vi "CH_LM Callback USBStreamingData.vi"(4 "User Parameter":variant, 5 "Event Data":T2, 6 "Control Ref":refnum<k7>, 7 "Event Common Data":T3) -> ()   [LabVIEW 2017, in "CH_LM.lvlib"]
doc: "This ActiveX callback VI is executed every time the corresponding ActiveX StreamData event occurs.\n\nThe event name together with the event data is written into a queue which is derived from a FGV (CH_SSIM Global Event Queues.vi). The queue is read from the CH_SSIM Streaming Read Data.vi.\n\n<B>Information:</B> ActiveX events with no corresponding combination of serial number and valid queue reference in the FGV are lost."
uses:
  CH_LM.lvlib
  CH_LM Event Cluster.ctl
  CH_LM Action Enumeration.ctl
  CH_LM_App/CH_LM Globals Debug-Status.vi
  CH_LM App.lvlib
panel:
  in  "CH_LM Event Cluster":T1
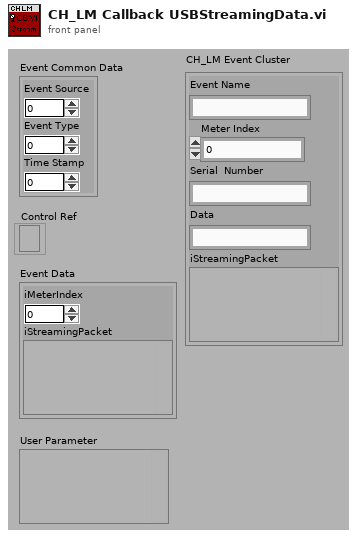
[diagram p1: front panel]
types:
  T1 = typedef "CH_LM.lvlib/CH_LM Event Cluster.ctl" = cluster{"Event Name":string, "Meter Index":i32, "Serial  Number":string, "Data":string, "iStreamingPacket":variant}
  T2 = cluster{"iMeterIndex":i16, "iStreamingPacket":variant}
  T3 = cluster{"Event Source":i32, "Event Type":u32, "Time Stamp":u32}
  T4 = typedef "CH_LM.lvlib/CH_LM Action Enumeration.ctl" = enum16{"add", "read", "read by serial", "set", "remove", "delete", "Clear Shift-Register", ""}
  T5 = typedef "CH_LM.lvlib/CH_LM Meter Info.ctl" = cluster{"Meter Index":i32, "Serial Number":string, "Queue Cluster":T6, "Data Header":bool, "Data Tokens":T7[]}
  T6 = typedef "CH_LM.lvlib/CH_LM Queue Cluster.ctl" = cluster{"Streaming Queue":refnum<queue>, "Asynch Notifier":refnum<notifier>}
  T7 = typedef "CH_LM.lvlib/CH_LM Data Token.ctl" = enum16{"Raw data", "Quad distance", "Formated data", "Unit", "Pulse period", "Flags", "Sequence ID"}
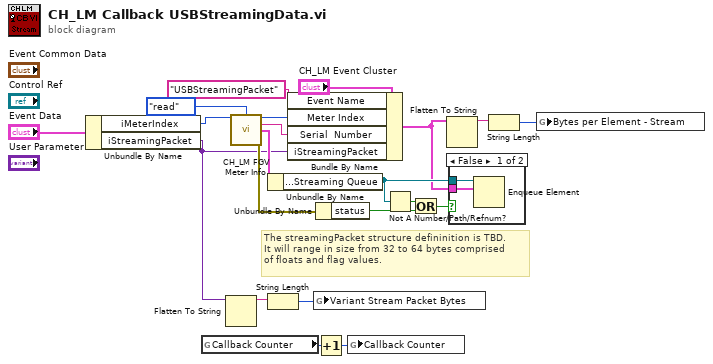
[diagram p0: block diagram]
diagram:
  # "The streamingPacket structure defininition is TBD.\nIt will range in size from 32 to 64 bytes comprised\nof floats and flag values."
  n1 = Unbundle By Name("Event Data") -> ("iMeterIndex"=w9:i16, "iStreamingPacket"=w8:variant)
  n2 = global read "CH_LM Globals Debug-Status.vi" "Callback Counter"() -> (w2:i32)
  n3 = Flatten To String(anything=w8) -> (data string=w7:string)  [unwired: 3 in, 2 out]
  n4 = call "CH_LM FGV Meter Info.vi"("Meter Index"=w9, "Action (read)"=CH_LM_Action_Enumeration."read") -> ("Meter Index out"=w12:i32, "Serial Number out"=w11:string, "Meter Info"=w19:T5, "error out"=w18:errorcluster)  [unwired: 3 in, 7 out]
  n5 = Unbundle By Name(w19) -> ("Queue Cluster.Streaming Queue"=w20:refnum<queue>)
  n6 = String Length(string=w7) -> (length=w6:i32)
  n7 = Bundle By Name(cluster="CH_LM Event Cluster", "Event Name"="USBStreamingPacket", "Meter Index"=w12, "Serial  Number"=w11, "iStreamingPacket"=w8) -> (w3:T1)
  n8 = global write "CH_LM Globals Debug-Status.vi" "Variant Stream Packet Bytes"(w6) -> ()
  n9 = Unbundle By Name(w18) -> ("status"=w14:bool)
  n10 = Increment(x=w2) -> (x+1=w1:i32)
  n11 = global write "CH_LM Globals Debug-Status.vi" "Callback Counter"(w1) -> ()
  n12 = Not A Number/Path/Refnum?(number/path/refnum=w20) -> (NaN/Path/Refnum?=w15:bool)
  n13 = Or(x=w15, y=w14) -> (x .or. y?=w13:bool)
  n14 = Flatten To String(anything=w3) -> (data string=w5:string)  [unwired: 3 in, 2 out]
  n15 = case shown="False" w13 {
    tunnel: w3 -> [w23 _]
    tunnel: w20 -> [w22 _]
    frame False {
      n16 = Enqueue Element(queue=w22, element=w23) -> ()  [unwired: 1 in, 4 out]
    }
    frame True {
    }
  }
  n17 = String Length(string=w5) -> (length=w4:i32)
  n18 = global write "CH_LM Globals Debug-Status.vi" "Bytes per Element - Stream"(w4) -> ()
